vi "CIFCore gRPC Test Client.vi"() -> ()   [LabVIEW 2021]
uses:
  Common/Typedef/Version.ctl
  Grpc/CIFCorePlugin_client/RPC Messages/cif_plugincore_PluginOverrides.ctl
  Grpc/CIFCorePlugin_client/RPC Messages/cif_plugincore_TimingOverrides.ctl
  Grpc/CIFCoreChannel_client/RPC Messages/cif_channelcore_FIFOInstance.ctl
  Common/Typedef/gRPC Reported Plugin Status.ctl
  Common/Typedef/Plugin State.ctl
  Common/Typedef/Timing Statistics.ctl
  Common/Typedef/Timing Stats Base.ctl
  Common/Typedef/FIFO Statistics.ctl
  Common/Typedef/Simple Error.ctl
  Common/Typedef/Monitor Doubles.ctl
  Common/Typedef/Monitor U64.ctl
  Common/Typedef/Monitor I64.ctl
  Grpc/CIFCoreChannel_client/RPC Messages/cif_channelcore_ConnectSubscriber.ctl
  Grpc/CIFCoreChannel_client/RPC Messages/cif_channelcore_ForceChannel.ctl
  <vilib>/gRPC/LabVIEW gRPC Library/Client API/Close Client.vi
  Grpc/CIFCoreWrapper/CIFCoreWrapper.lvlib
  Grpc/CIFCoreChannel_client/CIFCoreChannel_client.lvlib
  CIFUI/CIF_UI.lvclass
  Common/CIFCoreCommon.lvlib
  Grpc/CIFCorePlugin_client/CIFCorePlugin_client.lvlib
panel:
  out "Node Status":T1 {"Monitor Doubles"."4" format="%#_9g"; "Monitor Doubles"."3" format="%#_9g"; "Monitor Doubles"."2" format="%#_9g"; "Monitor Doubles"."1" format="%#_9g"; "Timing Statistics (us)"."Period"."Avg" format="%_6g"}
  in  "Clear Error":bool
  in  "Remove FIFO Instance":bool
  in  "instance_name":string
  out "new_instance_name":string
  in  "New FIFO Instance":T10
  in  "Add FIFO Instance":bool
  out "Plugin Names":T11
  in  "Channels":string(tree)
  in  "Force Channel":T12
  in  "force":bool
  in  "Connection":T13
  in  "connect":bool
  out "error out":errorcluster
  in  "JSON Configuration in":string
  in  "Quit":bool
  out "Plugin Overrides":T14
  out "Version":T16
  out "JSON Configuration":string
  in  "change config":bool
  in  "refresh":bool
  in  "stop":bool
  in  "pause":bool
  in  "start":bool
  in  "address":string="192.168.1.160:50051"
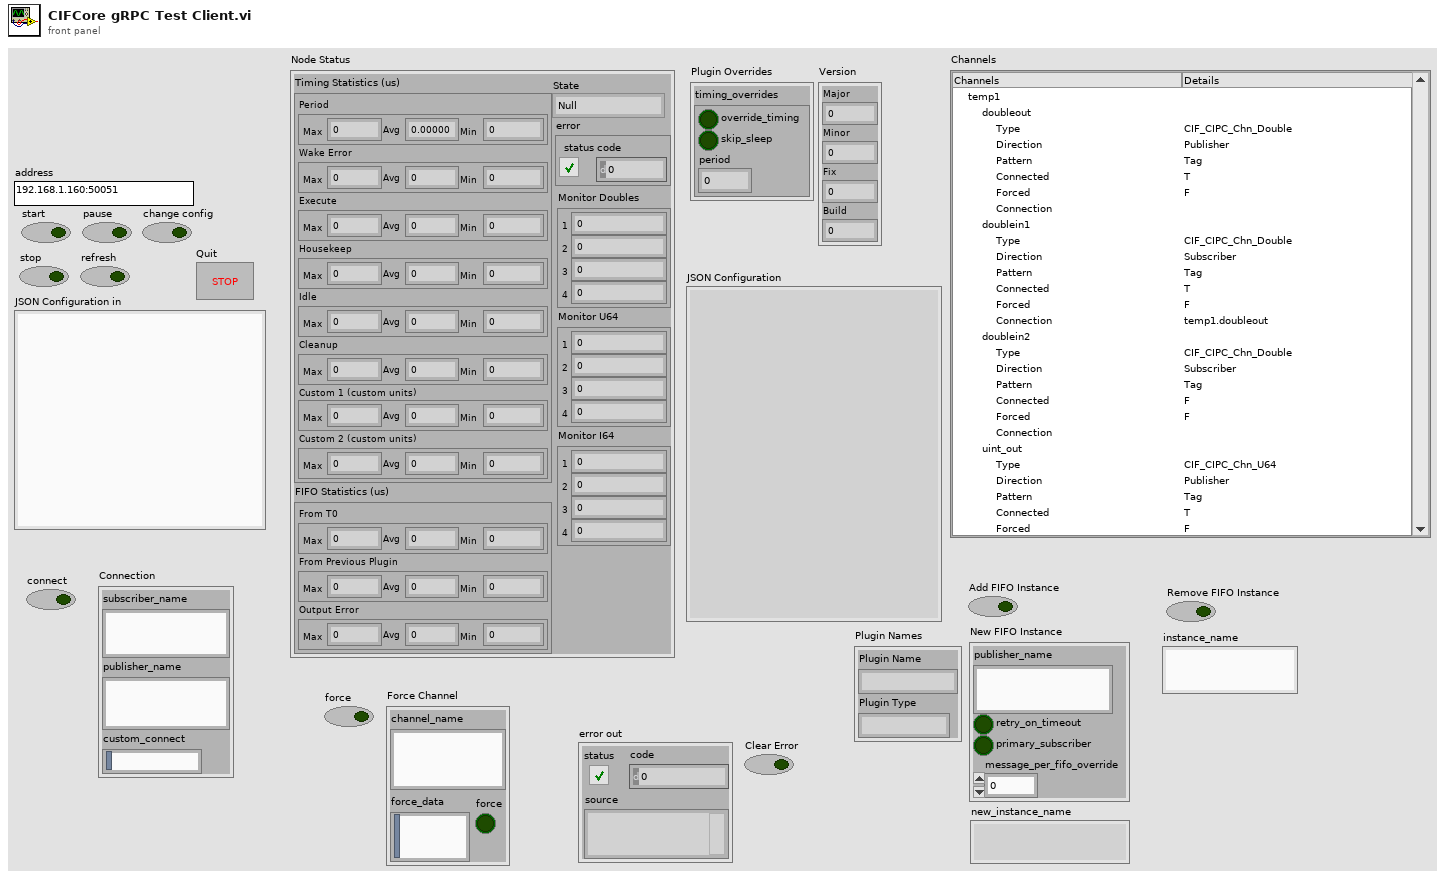
[diagram p1: front panel]
types:
  T1 = typedef "CIFCoreCommon.lvlib/gRPC Reported Plugin Status.ctl" = cluster{"State":T2, "Timing Statistics (us)":T3, "FIFO Statistics (us)":T5, "error":T6, "Monitor Doubles":T7, "Monitor U64":T8, "Monitor I64":T9}
  T2 = typedef "CIFCoreCommon.lvlib/Plugin State.ctl" = enum32{"Null", "Creating", "Listening", "Running", "CleaningUp", "Destroying"}
  T3 = typedef "CIFCoreCommon.lvlib/Timing Statistics.ctl" = cluster{"Period":T4, "Wake Error":T4, "Execute":T4, "Housekeep":T4, "Idle":T4, "Cleanup":T4, "Custom 1 (custom units)":T4, "Custom 2 (custom units)":T4}
  T4 = typedef "CIFCoreCommon.lvlib/Timing Stats Base.ctl" = cluster{"Max":i64, "Avg":dbl, "Min":i64}
  T5 = typedef "CIFCoreCommon.lvlib/FIFO Statistics.ctl" = cluster{"From T0":T4, "From Previous Plugin":T4, "Output Error":T4}
  T6 = typedef "CIFCoreCommon.lvlib/Simple Error.ctl" = cluster{"status":bool, "code":i32}
  T7 = typedef "CIFCoreCommon.lvlib/Monitor Doubles.ctl" = cluster{"1":dbl, "2":dbl, "3":dbl, "4":dbl}
  T8 = typedef "CIFCoreCommon.lvlib/Monitor U64.ctl" = cluster{"1":u64, "2":u64, "3":u64, "4":u64}
  T9 = typedef "CIFCoreCommon.lvlib/Monitor I64.ctl" = cluster{"1":i64, "2":i64, "3":i64, "4":i64}
  T10 = typedef "CIFCoreChannel_client.lvlib/cif_channelcore_FIFOInstance.ctl" = cluster{"publisher_name":string, "retry_on_timeout":bool, "primary_subscriber":bool, "message_per_fifo_override":u32}
  T11 = cluster{"Plugin Name":string, "Plugin Type":string}
  T12 = cluster{"channel_name":string, "force":bool, "force_data":string}
  T13 = cluster{"subscriber_name":string, "publisher_name":string, "custom_connect":string}
  T14 = typedef "CIFCorePlugin_client.lvlib/cif_plugincore_PluginOverrides.ctl" = cluster{"timing_overrides":T15}
  T15 = typedef "CIFCorePlugin_client.lvlib/cif_plugincore_TimingOverrides.ctl" = cluster{"override_timing":bool, "skip_sleep":bool, "period":dbl}
  T16 = typedef "CIFCoreCommon.lvlib/Version.ctl" = cluster{"Major":i32, "Minor":i32, "Fix":i32, "Build":i32}
  T17 = typedef "grpc-lvsupport-release.lvlib/grpcId.ctl" = u64
  T18 = typedef "CIFCoreChannel_client.lvlib/cif_channelcore_ConnectSubscriber.ctl" = cluster{"subscriber_name":string, "publisher_name":string, "custom_connect":u8[]}
  T19 = typedef "CIFCoreChannel_client.lvlib/cif_channelcore_ForceChannel.ctl" = cluster{"channel_name":string, "force":bool, "force_data":u8[]}
  T20 = typedef "CIFCoreChannel_client.lvlib/cif_channelcore_Channel.ctl" = cluster{"name":string, "direction":T21, "type":string, "custom_config":u8[], "connected":bool, "connected_name":string, "forced":bool, "channel_pattern":T22}
  T21 = typedef "CIFCoreChannel_client.lvlib/cif_channelcore_Direction.ctl" = enum32{"PUBLISHER", "SUBSCRIBER"}
  T22 = typedef "CIFCoreChannel_client.lvlib/cif_channelcore_PATTERN.ctl" = enum32{"UNKNOWN", "TAG", "FIFO", "MULTIFIFO"}
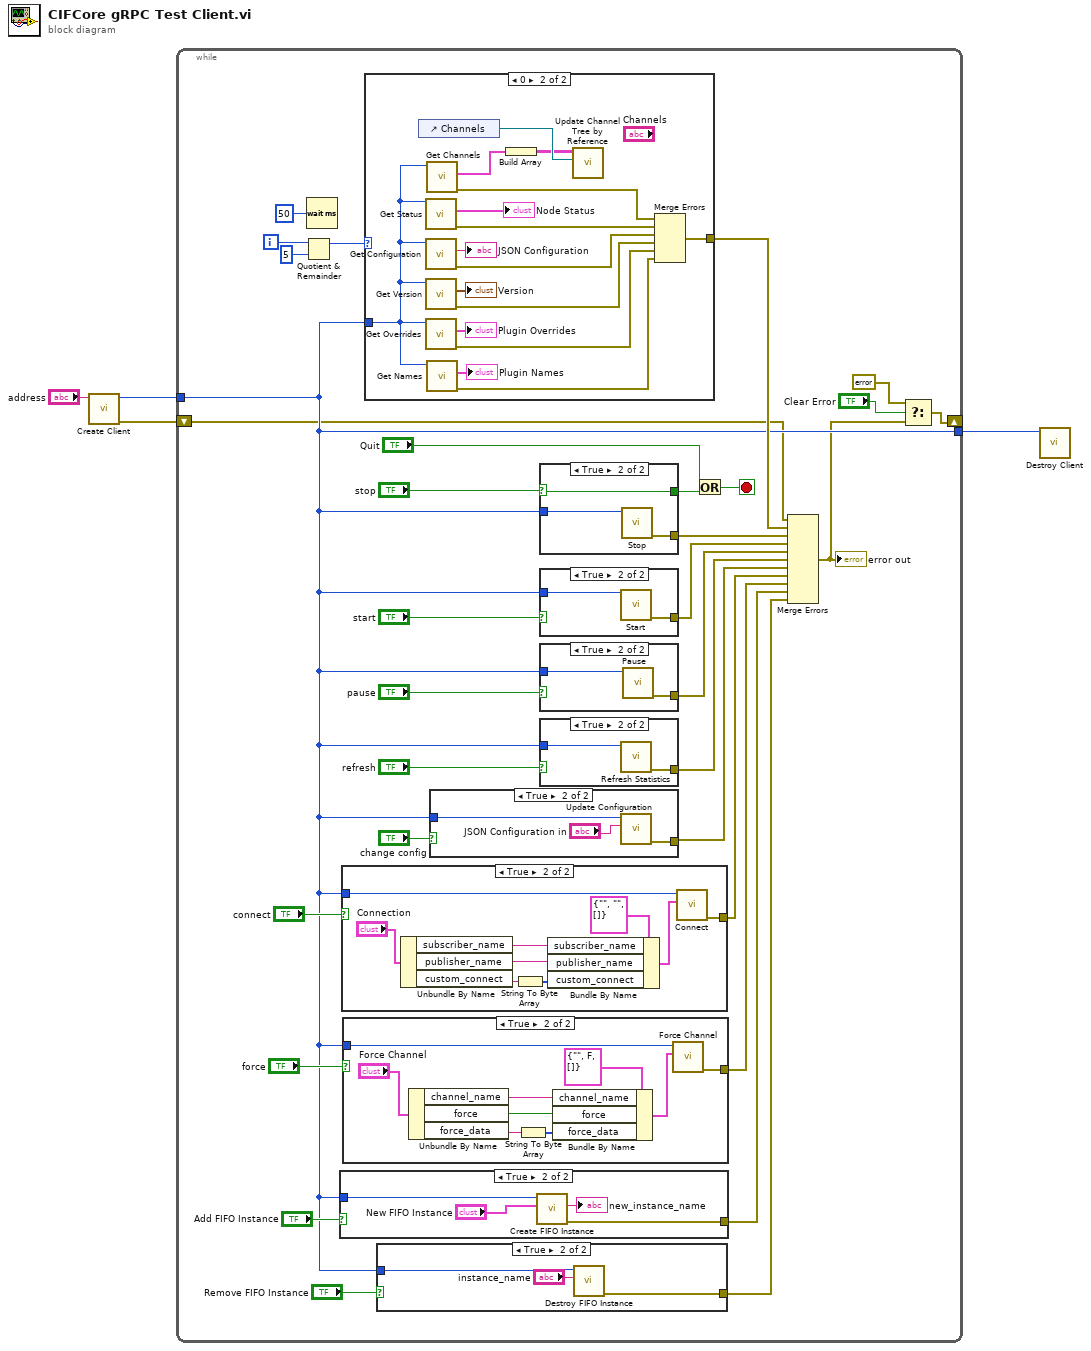
[diagram p0: block diagram]
diagram:
  n1 = call "Create Client.vi"("address"="address") -> ("error out"=w1:errorcluster, "gRPC ID Out"=w3:T17)  [unwired: 9 in]
  n2 = while {
    tunnel: w3 -> [w13]
    tunnel: [w13] -> w2
    shift-right: [w7] -> _
    shift-left: w1 -> [w9]
    i -> [w27]
    stop <- w29 stop-if-true
    n3 = Quotient & Remainder(x=w27, y=5) -> (x-y*floor(x/y)=w25:i32)  [unwired: 1 out]
    n4 = Wait (ms)(milliseconds to wait=u32 50) -> ()  [unwired: 1 out]
    n5 = case shown="True" "Add FIFO Instance" {
      tunnel: w13 -> [_ w43]
      tunnel: [_ w40] -> w12
      frame False {
      }
      frame True {
        n6 = call "Create FIFO Instance.vi"("New FIFO Instance"="New FIFO Instance", "gRPC ID"=w43) -> ("error out"=w40:errorcluster, "publisher_instance_name"=→"new_instance_name":string)  [unwired: 7 in, 1 out]
      }
    }
    n7 = case shown="True" "connect" {
      tunnel: w13 -> [_ w47]
      tunnel: [_ w48] -> w16
      frame False {
      }
      frame True {
        n8 = Unbundle By Name("Connection") -> ("subscriber_name"=w52:string, "publisher_name"=w51:string, "custom_connect"=w49:string)
        n9 = String To Byte Array(string=w49) -> (unsigned byte array=w50:u8[])
        n10 = Bundle By Name(cluster=T18 {"subscriber_name"="", "publisher_name"="", "custom_connect"=[]} ("Connection 2"), "subscriber_name"=w52, "publisher_name"=w51, "custom_connect"=w50) -> (w44:T18)
        n11 = call "Connect.vi"("Connection"=w44, "gRPC ID"=w47) -> ("error out"=w48:errorcluster)  [unwired: 8 in, 1 out]
      }
    }
    n12 = case shown="True" "force" {
      tunnel: w13 -> [_ w61]
      tunnel: [_ w60] -> w17
      frame False {
      }
      frame True {
        n13 = Unbundle By Name("Force Channel") -> ("channel_name"=w59:string, "force"=w56:bool, "force_data"=w54:string)
        n14 = String To Byte Array(string=w54) -> (unsigned byte array=w55:u8[])
        n15 = Bundle By Name(cluster=T19 {"channel_name"="", "force"=FALSE, "force_data"=[]} ("Force Channel"), "channel_name"=w59, "force"=w56, "force_data"=w55) -> (w57:T19)
        n16 = call "Force Channel.vi"("Force Channel"=w57, "gRPC ID"=w61) -> ("error out"=w60:errorcluster)  [unwired: 8 in, 1 out]
      }
    }
    n17 = case shown="0" w25 {
      tunnel: w13 -> [_ w67]
      tunnel: [_ w70] -> w19
      frame 1, Default {
      }
      frame 0 {
        n18 = control-ref of="Channels"() -> (w64:refnum<vi>)
        n19 = call "Get Status.vi"("gRPC ID"=w67) -> ("error out"=w74:errorcluster, "Node Status"=→"Node Status":T1)  [unwired: 8 in, 1 out]
        n20 = call "Get Configuration.vi"("gRPC ID"=w67) -> ("error out"=w73:errorcluster, "JSON Configuration"=→"JSON Configuration":string)  [unwired: 8 in, 1 out]
        n21 = call "Get Version.vi"("gRPC ID"=w67) -> ("error out"=w72:errorcluster, "Version"=→"Version":T16)  [unwired: 8 in, 1 out]
        n22 = call "Get Overrides.vi"("gRPC ID"=w67) -> ("error out"=w71:errorcluster, "Plugin Overrides"=→"Plugin Overrides":T14)  [unwired: 8 in, 1 out]
        n23 = call "Get Channels.vi"("gRPC ID"=w67) -> ("error out"=w69:errorcluster, "Channels"=w68:T20[])  [unwired: 8 in, 1 out]
        n24 = call "Get Names.vi"("gRPC ID"=w67) -> ("error out"=w65:errorcluster, "Plugin Names"=→"Plugin Names":T11)  [unwired: 8 in, 1 out]
        n25 = Build Array(w68) -> (w63:T20[][])
        n26 = call "Update Channel Tree by Reference.vi"("Channnel Tree ref in"=w64, "Channels"=w63) -> ()  [unwired: 9 in, 1 out]
        n27 = Merge Errors(w69, w74, w73, w72, w71, w65) -> (w70:errorcluster)
      }
    }
    n28 = case shown="True" "Remove FIFO Instance" {
      tunnel: w13 -> [_ w39]
      tunnel: [_ w37] -> w11
      frame False {
      }
      frame True {
        n29 = call "Destroy FIFO Instance.vi"("publisher_instance_name"="instance_name", "gRPC ID"=w39) -> ("error out"=w37:errorcluster)  [unwired: 8 in, 1 out]
      }
    }
    n30 = case shown="True" "change config" {
      tunnel: w13 -> [_ w80]
      tunnel: [_ w78] -> w20
      frame False {
      }
      frame True {
        n31 = call "Update Configuration.vi"("JSON Configuration"="JSON Configuration in", "gRPC ID"=w80) -> ("error out"=w78:errorcluster)  [unwired: 8 in, 1 out]
      }
    }
    n32 = case shown="True" "stop" {
      selector: "stop" -> [_ w84]
      tunnel: w13 -> [_ w85]
      tunnel: [_ w84] -> w28
      tunnel: [_ w83] -> w24
      frame False {
      }
      frame True {
        n33 = call "Stop.vi"("gRPC ID"=w85) -> ("error out"=w83:errorcluster)  [unwired: 9 in, 1 out]
      }
    }
    n34 = case shown="True" "start" {
      tunnel: w13 -> [_ w89]
      tunnel: [_ w88] -> w23
      frame False {
      }
      frame True {
        n35 = call "Start.vi"("gRPC ID"=w89) -> ("error out"=w88:errorcluster)  [unwired: 9 in, 1 out]
      }
    }
    n36 = case shown="True" "pause" {
      tunnel: w13 -> [_ w87]
      tunnel: [_ w86] -> w22
      frame False {
      }
      frame True {
        n37 = call "Pause.vi"("gRPC ID"=w87) -> ("error out"=w86:errorcluster)  [unwired: 9 in, 1 out]
      }
    }
    n38 = case shown="True" "refresh" {
      tunnel: w13 -> [_ w82]
      tunnel: [_ w81] -> w21
      frame False {
      }
      frame True {
        n39 = call "Refresh Statistics.vi"("gRPC ID"=w82) -> ("error out"=w81:errorcluster)  [unwired: 9 in, 1 out]
      }
    }
    n40 = Or(x="Quit", y=w28) -> (x .or. y?=w29:bool)
    n41 = Merge Errors(w9, w19, w24, w23, w22, w21, w20, w16, w17, w12, w11) -> (w8:errorcluster)
    "error out" <- w8
    n42 = Select(t=errorcluster {"status"=FALSE, "code"=0, "source"=""}, s="Clear Error", f=w8) -> (s? t:f=w7:errorcluster)
  }
  n43 = call "Destroy Client.vi"("gRPC ID"=w2) -> ()  [unwired: 10 in, 1 out]
